vi "bundle_ai_for_clock_transfer.vi"(8 "FIFO Refs":T1={"FIFO 0"="AI Bundel FIFO 0", "FIFO 1"="AI Bundel FIFO 1", "FIFO 2"="AI Bundel FIFO 2", "FIFO 3"="AI Bundel FIFO 3", "FIFO 4"="AI Bundel FIFO 4", "FIFO 5"="AI Bundel FIFO 5", "FIFO 6"="AI Bundel FIFO 6", "FIFO 7"="AI Bundel FIFO 7"}, 9 "sample":i16, 10 "Debug":bool, 11 "Input Valid":bool) -> (3 "Ready for Input":bool)   [LabVIEW 2014]
doc: "Aquire 32 channels of analog input and bundle channels as groups of 4 into FIFOs.\nOptionally a debug true can be passed which generates data for each analog channel to produce an offset line with slope one for debugging purposes."
uses:
  FPGA_Controls/Acquisition FIFOs Cluster.ctl
  <vilib>/rvi/eio/common/nirviEmuTemplateMethod_errors.vi
  <vilib>/eio/EIONode/EIONode.xnode
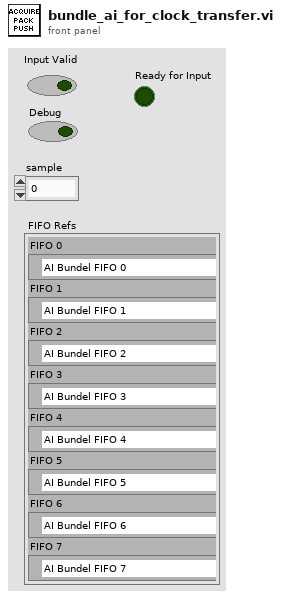
[diagram p1: front panel]
types:
  T1 = typedef "Acquisition FIFOs Cluster.ctl" = cluster{"FIFO 0":refnum<k21>, "FIFO 1":refnum<k21>, "FIFO 2":refnum<k21>, "FIFO 3":refnum<k21>, "FIFO 4":refnum<k21>, "FIFO 5":refnum<k21>, "FIFO 6":refnum<k21>, "FIFO 7":refnum<k21>}
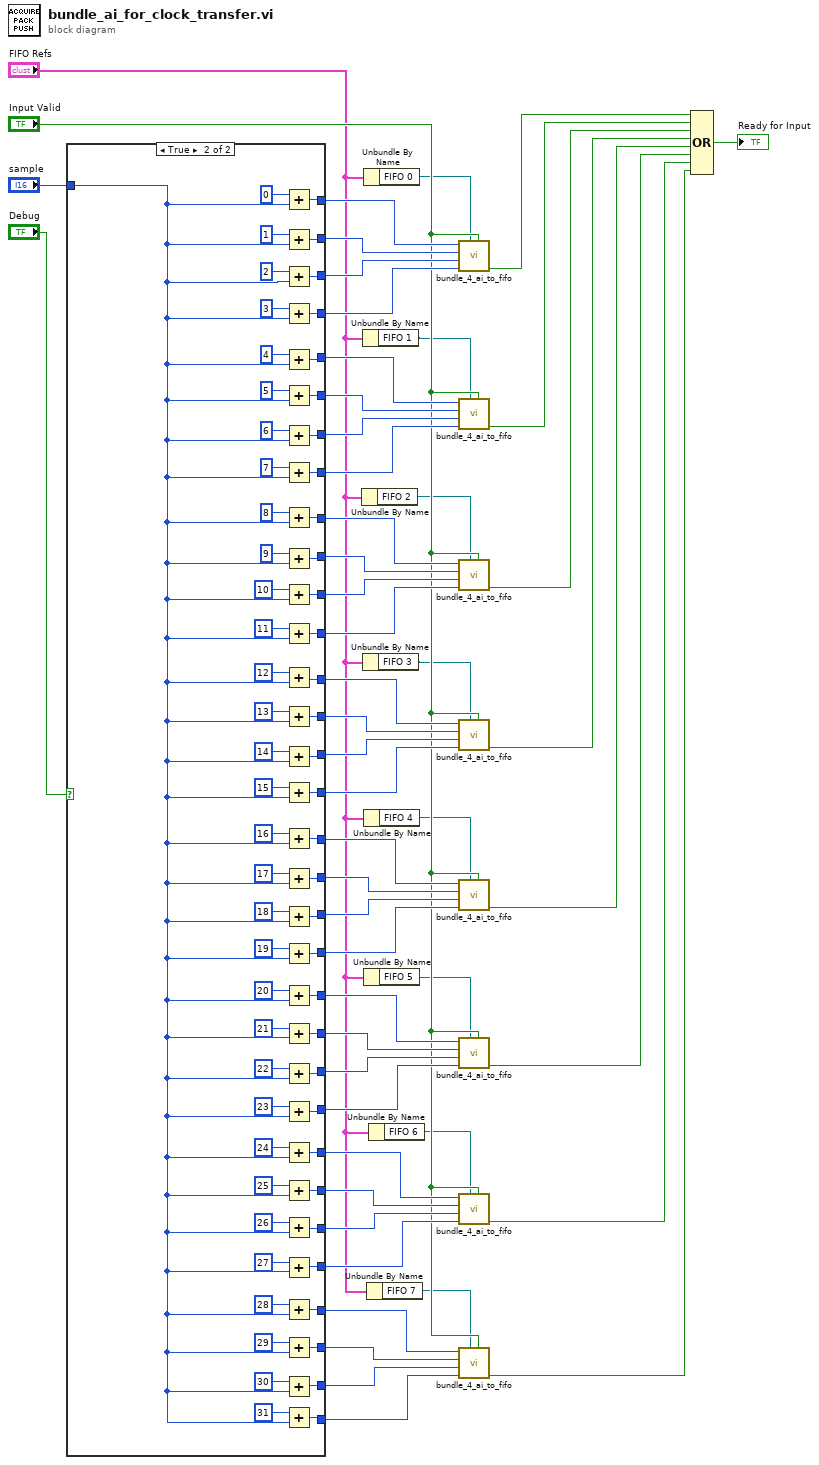
[diagram p0: block diagram]
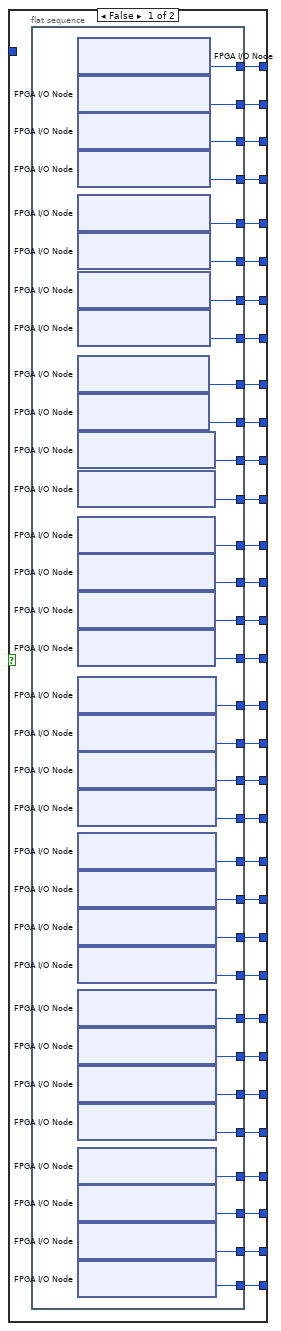
[diagram p2: hidden frame]
diagram:
  n1 = case shown="True" "Debug" {
    tunnel: [w85 w182] -> w52
    tunnel: [w84 w179] -> w51
    tunnel: [w83 w177] -> w50
    tunnel: [w82 w175] -> w49
    tunnel: [w81 w173] -> w48
    tunnel: [w80 w171] -> w47
    tunnel: [w79 w169] -> w46
    tunnel: [w78 w167] -> w45
    tunnel: [w77 w163] -> w44
    tunnel: [w76 w162] -> w43
    tunnel: [w75 w161] -> w42
    tunnel: [w74 w159] -> w41
    tunnel: [w73 w157] -> w40
    tunnel: [w72 w151] -> w39
    tunnel: [w71 w155] -> w38
    tunnel: [w70 w153] -> w37
    tunnel: [w69 w149] -> w36
    tunnel: [w68 w147] -> w35
    tunnel: [w67 w145] -> w34
    tunnel: [w66 w143] -> w33
    tunnel: [w65 w141] -> w32
    tunnel: [w64 w139] -> w31
    tunnel: [w63 w137] -> w30
    tunnel: [w62 w135] -> w29
    tunnel: [w61 w133] -> w28
    tunnel: [w60 w127] -> w27
    tunnel: [w59 w131] -> w26
    tunnel: [w58 w129] -> w25
    tunnel: [w57 w125] -> w24
    tunnel: [w56 w123] -> w23
    tunnel: [w55 w121] -> w22
    tunnel: [w54 w119] -> w21
    tunnel: "sample" -> [_ w118]
    frame False {
      n2 = flat-sequence {
        tunnel: [w117] -> w85
        tunnel: [w116] -> w84
        tunnel: [w115] -> w83
        tunnel: [w114] -> w82
        tunnel: [w113] -> w81
        tunnel: [w112] -> w80
        tunnel: [w111] -> w79
        tunnel: [w110] -> w78
        tunnel: [w109] -> w77
        tunnel: [w108] -> w76
        tunnel: [w107] -> w75
        tunnel: [w106] -> w74
        tunnel: [w105] -> w73
        tunnel: [w104] -> w71
        tunnel: [w103] -> w70
        tunnel: [w102] -> w72
        tunnel: [w101] -> w54
        tunnel: [w100] -> w55
        tunnel: [w99] -> w56
        tunnel: [w98] -> w57
        tunnel: [w97] -> w60
        tunnel: [w96] -> w58
        tunnel: [w95] -> w59
        tunnel: [w94] -> w61
        tunnel: [w93] -> w62
        tunnel: [w92] -> w63
        tunnel: [w91] -> w64
        tunnel: [w90] -> w65
        tunnel: [w89] -> w66
        tunnel: [w88] -> w67
        tunnel: [w87] -> w68
        tunnel: [w86] -> w69
        frame #0 {
          n3 = xnode "FPGA I/O Node"() -> ("IO Module\\AI A0"=w117:i16)  [unwired: 1 in, 1 out]
          n4 = xnode "FPGA I/O Node"() -> ("IO Module\\AI A1"=w116:i16)  [unwired: 1 in, 1 out]
          n5 = xnode "FPGA I/O Node"() -> ("IO Module\\AI A2"=w115:i16)  [unwired: 1 in, 1 out]
          n6 = xnode "FPGA I/O Node"() -> ("IO Module\\AI A3"=w114:i16)  [unwired: 1 in, 1 out]
          n7 = xnode "FPGA I/O Node"() -> ("IO Module\\AI A4"=w113:i16)  [unwired: 1 in, 1 out]
          n8 = xnode "FPGA I/O Node"() -> ("IO Module\\AI A5"=w112:i16)  [unwired: 1 in, 1 out]
          n9 = xnode "FPGA I/O Node"() -> ("IO Module\\AI A6"=w111:i16)  [unwired: 1 in, 1 out]
          n10 = xnode "FPGA I/O Node"() -> ("IO Module\\AI A7"=w110:i16)  [unwired: 1 in, 1 out]
          n11 = xnode "FPGA I/O Node"() -> ("IO Module\\AI B8"=w109:i16)  [unwired: 1 in, 1 out]
          n12 = xnode "FPGA I/O Node"() -> ("IO Module\\AI B9"=w108:i16)  [unwired: 1 in, 1 out]
          n13 = xnode "FPGA I/O Node"() -> ("IO Module\\AI B10"=w107:i16)  [unwired: 1 in, 1 out]
          n14 = xnode "FPGA I/O Node"() -> ("IO Module\\AI B11"=w106:i16)  [unwired: 1 in, 1 out]
          n15 = xnode "FPGA I/O Node"() -> ("IO Module\\AI B12"=w105:i16)  [unwired: 1 in, 1 out]
          n16 = xnode "FPGA I/O Node"() -> ("IO Module\\AI B13"=w104:i16)  [unwired: 1 in, 1 out]
          n17 = xnode "FPGA I/O Node"() -> ("IO Module\\AI B14"=w103:i16)  [unwired: 1 in, 1 out]
          n18 = xnode "FPGA I/O Node"() -> ("IO Module\\AI B15"=w102:i16)  [unwired: 1 in, 1 out]
          n19 = xnode "FPGA I/O Node"() -> ("IO Module\\AI C16"=w86:i16)  [unwired: 1 in, 1 out]
          n20 = xnode "FPGA I/O Node"() -> ("IO Module\\AI C17"=w87:i16)  [unwired: 1 in, 1 out]
          n21 = xnode "FPGA I/O Node"() -> ("IO Module\\AI C18"=w88:i16)  [unwired: 1 in, 1 out]
          n22 = xnode "FPGA I/O Node"() -> ("IO Module\\AI C19"=w89:i16)  [unwired: 1 in, 1 out]
          n23 = xnode "FPGA I/O Node"() -> ("IO Module\\AI C20"=w90:i16)  [unwired: 1 in, 1 out]
          n24 = xnode "FPGA I/O Node"() -> ("IO Module\\AI C21"=w91:i16)  [unwired: 1 in, 1 out]
          n25 = xnode "FPGA I/O Node"() -> ("IO Module\\AI C22"=w92:i16)  [unwired: 1 in, 1 out]
          n26 = xnode "FPGA I/O Node"() -> ("IO Module\\AI C23"=w93:i16)  [unwired: 1 in, 1 out]
          n27 = xnode "FPGA I/O Node"() -> ("IO Module\\AI D24"=w94:i16)  [unwired: 1 in, 1 out]
          n28 = xnode "FPGA I/O Node"() -> ("IO Module\\AI D25"=w95:i16)  [unwired: 1 in, 1 out]
          n29 = xnode "FPGA I/O Node"() -> ("IO Module\\AI D26"=w96:i16)  [unwired: 1 in, 1 out]
          n30 = xnode "FPGA I/O Node"() -> ("IO Module\\AI D27"=w97:i16)  [unwired: 1 in, 1 out]
          n31 = xnode "FPGA I/O Node"() -> ("IO Module\\AI D28"=w98:i16)  [unwired: 1 in, 1 out]
          n32 = xnode "FPGA I/O Node"() -> ("IO Module\\AI D29"=w99:i16)  [unwired: 1 in, 1 out]
          n33 = xnode "FPGA I/O Node"() -> ("IO Module\\AI D30"=w100:i16)  [unwired: 1 in, 1 out]
          n34 = xnode "FPGA I/O Node"() -> ("IO Module\\AI D31"=w101:i16)  [unwired: 1 in, 1 out]
        }
      }
    }
    frame True {
      n35 = Add(x=i16 0, y=w118) -> (x+y=w182:i16)
      n36 = Add(x=i16 1, y=w118) -> (x+y=w179:i16)
      n37 = Add(x=i16 2, y=w118) -> (x+y=w177:i16)
      n38 = Add(x=i16 3, y=w118) -> (x+y=w175:i16)
      n39 = Add(x=i16 4, y=w118) -> (x+y=w173:i16)
      n40 = Add(x=i16 5, y=w118) -> (x+y=w171:i16)
      n41 = Add(x=i16 6, y=w118) -> (x+y=w169:i16)
      n42 = Add(x=i16 7, y=w118) -> (x+y=w167:i16)
      n43 = Add(x=i16 8, y=w118) -> (x+y=w163:i16)
      n44 = Add(x=i16 9, y=w118) -> (x+y=w162:i16)
      n45 = Add(x=i16 10, y=w118) -> (x+y=w161:i16)
      n46 = Add(x=i16 11, y=w118) -> (x+y=w159:i16)
      n47 = Add(x=i16 12, y=w118) -> (x+y=w157:i16)
      n48 = Add(x=i16 13, y=w118) -> (x+y=w155:i16)
      n49 = Add(x=i16 14, y=w118) -> (x+y=w153:i16)
      n50 = Add(x=i16 15, y=w118) -> (x+y=w151:i16)
      n51 = Add(x=i16 16, y=w118) -> (x+y=w149:i16)
      n52 = Add(x=i16 17, y=w118) -> (x+y=w147:i16)
      n53 = Add(x=i16 18, y=w118) -> (x+y=w145:i16)
      n54 = Add(x=i16 19, y=w118) -> (x+y=w143:i16)
      n55 = Add(x=i16 20, y=w118) -> (x+y=w141:i16)
      n56 = Add(x=i16 21, y=w118) -> (x+y=w139:i16)
      n57 = Add(x=i16 22, y=w118) -> (x+y=w137:i16)
      n58 = Add(x=i16 23, y=w118) -> (x+y=w135:i16)
      n59 = Add(x=i16 24, y=w118) -> (x+y=w133:i16)
      n60 = Add(x=i16 25, y=w118) -> (x+y=w131:i16)
      n61 = Add(x=i16 26, y=w118) -> (x+y=w129:i16)
      n62 = Add(x=i16 27, y=w118) -> (x+y=w127:i16)
      n63 = Add(x=i16 28, y=w118) -> (x+y=w125:i16)
      n64 = Add(x=i16 29, y=w118) -> (x+y=w123:i16)
      n65 = Add(x=i16 30, y=w118) -> (x+y=w121:i16)
      n66 = Add(x=i16 31, y=w118) -> (x+y=w119:i16)
    }
  }
  n67 = Unbundle By Name("FIFO Refs") -> ("FIFO 2"=w9:refnum<k21>)
  n68 = Unbundle By Name("FIFO Refs") -> ("FIFO 1"=w10:refnum<k21>)
  n69 = Unbundle By Name("FIFO Refs") -> ("FIFO 3"=w8:refnum<k21>)
  n70 = Unbundle By Name("FIFO Refs") -> ("FIFO 0"=w11:refnum<k21>)
  n71 = Unbundle By Name("FIFO Refs") -> ("FIFO 4"=w7:refnum<k21>)
  n72 = Unbundle By Name("FIFO Refs") -> ("FIFO 5"=w4:refnum<k21>)
  n73 = Unbundle By Name("FIFO Refs") -> ("FIFO 7"=w6:refnum<k21>)
  n74 = Unbundle By Name("FIFO Refs") -> ("FIFO 6"=w5:refnum<k21>)
  n75 = call "bundle_4_ai_to_fifo.vi"("Input Valid"="Input Valid", "FIFO In"=w11, "AI3"=w49, "AI2"=w50, "AI1"=w51, "AI0"=w52) -> ("Ready for Input"=w12:bool)  [unwired: 5 in]
  n76 = call "bundle_4_ai_to_fifo.vi"("Input Valid"="Input Valid", "FIFO In"=w10, "AI3"=w45, "AI2"=w46, "AI1"=w47, "AI0"=w48) -> ("Ready for Input"=w13:bool)  [unwired: 5 in]
  n77 = call "bundle_4_ai_to_fifo.vi"("Input Valid"="Input Valid", "FIFO In"=w9, "AI3"=w41, "AI2"=w42, "AI1"=w43, "AI0"=w44) -> ("Ready for Input"=w14:bool)  [unwired: 5 in]
  n78 = call "bundle_4_ai_to_fifo.vi"("Input Valid"="Input Valid", "FIFO In"=w8, "AI3"=w39, "AI2"=w37, "AI1"=w38, "AI0"=w40) -> ("Ready for Input"=w15:bool)  [unwired: 5 in]
  n79 = call "bundle_4_ai_to_fifo.vi"("Input Valid"="Input Valid", "FIFO In"=w7, "AI3"=w33, "AI2"=w34, "AI1"=w35, "AI0"=w36) -> ("Ready for Input"=w16:bool)  [unwired: 5 in]
  n80 = call "bundle_4_ai_to_fifo.vi"("Input Valid"="Input Valid", "FIFO In"=w4, "AI3"=w29, "AI2"=w30, "AI1"=w31, "AI0"=w32) -> ("Ready for Input"=w17:bool)  [unwired: 5 in]
  n81 = call "bundle_4_ai_to_fifo.vi"("Input Valid"="Input Valid", "FIFO In"=w5, "AI3"=w27, "AI2"=w25, "AI1"=w26, "AI0"=w28) -> ("Ready for Input"=w18:bool)  [unwired: 5 in]
  n82 = call "bundle_4_ai_to_fifo.vi"("Input Valid"="Input Valid", "FIFO In"=w6, "AI3"=w21, "AI2"=w22, "AI1"=w23, "AI0"=w24) -> ("Ready for Input"=w19:bool)  [unwired: 5 in]
  n83 = Compound Arithmetic op=OR(w12, w13, w14, w15, w16, w17, w18, w19) -> (→"Ready for Input":bool)
